vi "KKT_matrix_11.vi"(1 "lmd_input":dbl[](array[numeric]), 2 "constraints cluster":T2, 3 "Object cluster":T3) -> (0 "KKT_matrix_11":T1)   [LabVIEW 2019]
uses:
  <vilib>/Analysis/Matrix/Datatypes/RealMatrix.ctl
  <vilib>/Analysis/Matrix/Numeric/Conversions/Array To Matrix - RA2.vi
  <vilib>/Analysis/Matrix/NI_Matrix.lvlib
panel:
  # "input : object cluster\n             constraints cluster\n             lmd_input"
  # "output : KKT_matrix_11, \n               n*n"
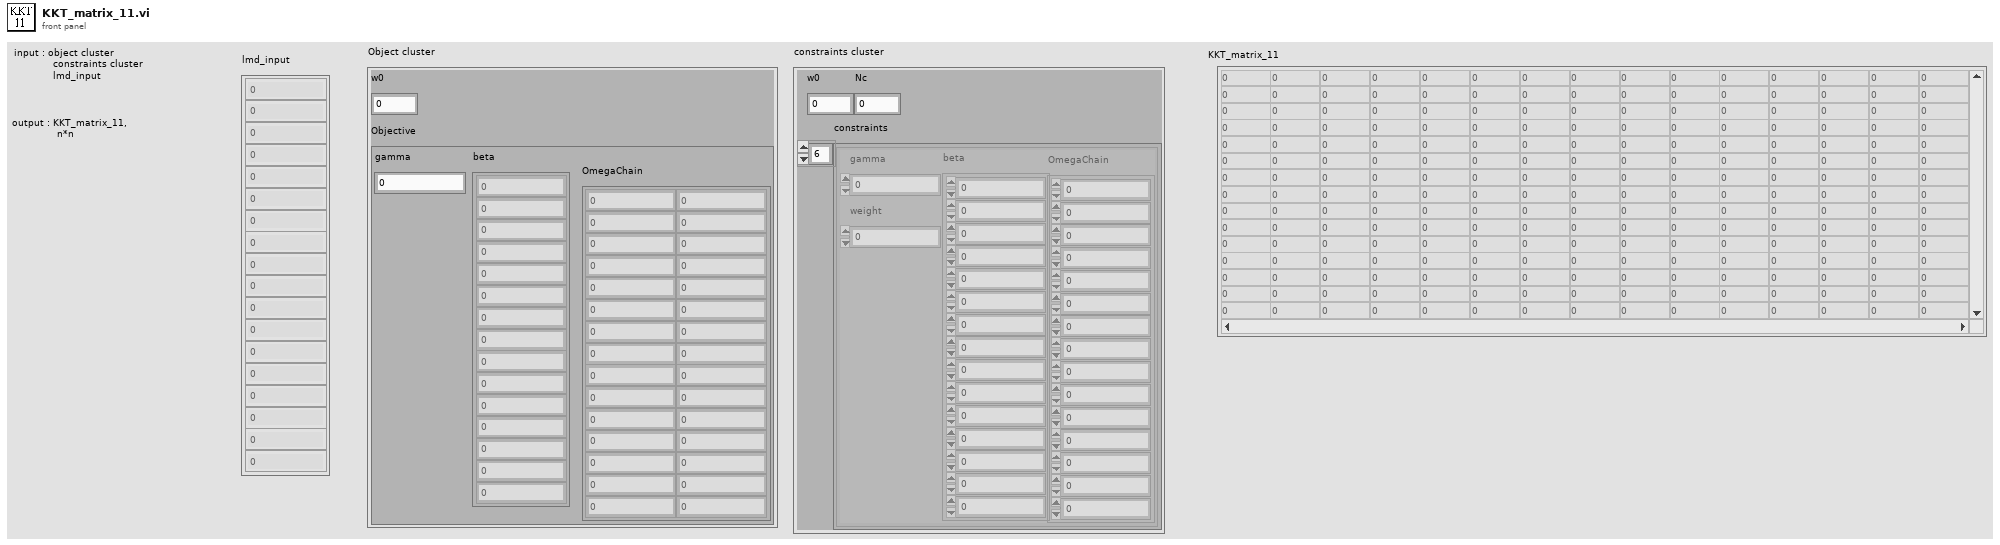
[diagram p1: front panel]
types:
  T1 = typedef "NI_Matrix.lvlib/RealMatrix.ctl" = dbl[][]
  T2 = cluster{"w0":dbl, "constraints":cluster{"beta":dbl[], "gamma":dbl, "OmegaChain":dbl[], "weight":dbl}[], "Nc":i32}
  T3 = cluster{"w0":dbl, "Objective":cluster{"beta":dbl[], "gamma":dbl, "OmegaChain":dbl[][]}}
  T4 = cluster{"beta":dbl[], "gamma":dbl, "OmegaChain":dbl[][]}
  T5 = cluster{"beta":dbl[], "gamma":dbl, "OmegaChain":dbl[], "weight":dbl}[]
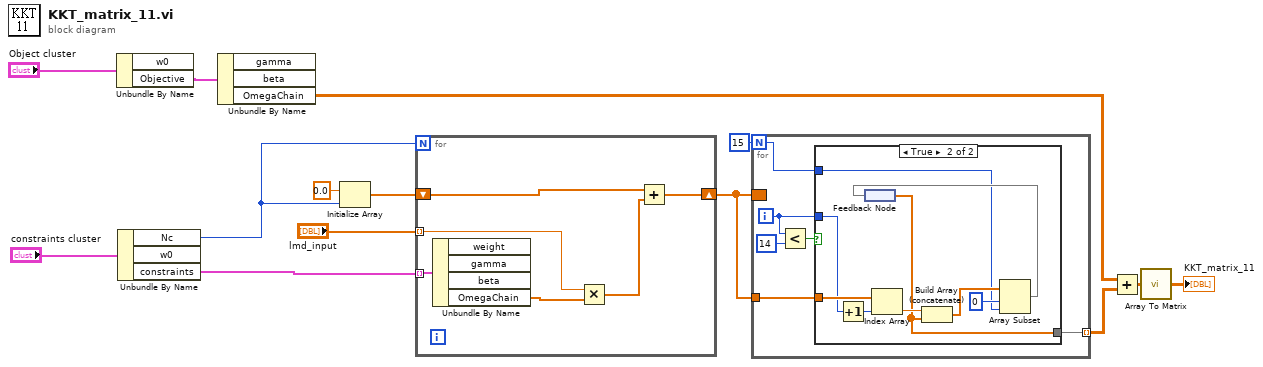
[diagram p0: block diagram]
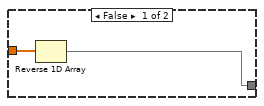
[diagram p2: hidden frame]
diagram:
  n1 = Unbundle By Name("Object cluster") -> ("Objective"=w12:T4)  [unwired: 1 out]
  n2 = Unbundle By Name("constraints cluster") -> ("Nc"=w7:i32, "constraints"=w10:T5)  [unwired: 1 out]
  n3 = Unbundle By Name(w12) -> ("OmegaChain"=w5:dbl[][])  [unwired: 2 out]
  n4 = Initialize Array(0.0 ("element"), w7) -> (w8:dbl[])
  n5 = for {
    N: w7 -> [_]
    tunnel: "lmd_input" -> [w19] mode=indexing
    tunnel: w10 -> [w20] mode=indexing
    shift-right: [w15] -> w1
    shift-left: w8 -> [w17]
    n6 = Unbundle By Name(w20) -> ("OmegaChain"=w18:dbl[])  [unwired: 3 out]
    n7 = Multiply(x=w19, y=w18) -> (x*y=w16:dbl[])
    n8 = Add(x=w17, y=w16) -> (x+y=w15:dbl[])
  }
  n9 = for {
    N: 15 -> [w21]
    tunnel: [w22] -> w6 mode=indexing
    border: w1 -> [_]
    tunnel: w1 -> [w26]
    i -> [w23]
    n10 = Less?(x=w23, y=14) -> (x < y?=w24:bool)
    n11 = case shown="True" w24 {
      tunnel: w26 -> [w28 w35]
      tunnel: w23 -> [_ w32]
      tunnel: [w27 w30] -> w22
      tunnel: w21 -> [_ w29]
      frame False {
        n12 = Reverse 1D Array(array=w28) -> (reversed array=w27:dbl[])
      }
      frame True {
        n13 = Increment(x=w32) -> (x+1=w33:i32)
        n14 = feedback #1() -> (w30:dbl[])
        n15 = Index Array(array=w35, index=w33) -> (element=w34:dbl)
        n16 = Build Array (concatenate)(w34, w30) -> (w36:dbl[])
        n17 = Array Subset(array=w36, index=0, length=w29) -> (w31:dbl[])
        n18 = feedback-in #1(w31) -> ()
      }
    }
  }
  n19 = Add(x=w5, y=w6) -> (x+y=w4:dbl[][])
  n20 = call-poly <vilib>:"Array To Matrix.vi"("Real 2D Array"=w4) -> ("Real Matrix"=→"KKT_matrix_11":T1)
